vi "Autonomous Independent.vi"   [LabVIEW 2012]
doc: "This VI is called when autonomous begins, and will automatically be terminated when autonomous ends. You can carry out timed or sensor driven robot movement independently without needing to return to the caller."
uses:
  <vilib>/Rock Robotics/WPI/Joystick/WPI_JoystickGetSetRefNum.vi
  Robot Global Data.vi
  <vilib>/Rock Robotics/WPI/RobotDrive/WPI_RobotDriveMecanumDrive_Cartesian.vi
  <vilib>/Rock Robotics/WPI/Solenoid/WPI_SolenoidValue.ctl
  <vilib>/Rock Robotics/WPI/Solenoid/WPI_SolenoidSetEnum.vi
  SubVI/Global 1 (shooter controls).vi
panel:
  # "Be sure to right-click and choose Data Operations>>Make Current Value default if you want to save the array values with the VI"
types:
  T1 = typedef "WPI_SolenoidValue.ctl" = enum16{"Off", "On", "Forward", "Reverse"}
  T2 = enum16{"fire only", "comlex fire 5", "slide left fire", "slide right fire"}
  T3 = typedef "WPI_SolenoidDevRef.ctl" = cluster{"DevStatus":errorcluster, "Solenoid Module":T4, "Forward Solenoid Channel":T5, "Reverse Solenoid Channel":T5}
  T4 = typedef "FPGA_TypedefSolenoidModule.ctl" = enum16{"Solenoid Module 1", "Solenoid Module 2"}
  T5 = typedef "WPI_SolenoidChannel.ctl" = enum8{"Solenoid 1", "Solenoid 2", "Solenoid 3", "Solenoid 4", "Solenoid 5", "Solenoid 6", "Solenoid 7", "Solenoid 8", "Invalid"}
  T6 = typedef "WPI_RobotDriveDevRef.ctl" = cluster{"DevStatus":errorcluster, "Motors[]":T7[], "Square Inputs":bool, "Max Output":dbl, "Isochronous":bool}
  T7 = typedef "WPI_MotorControlDeviceRef.ctl" = cluster{"DeviceStatus":errorcluster, "Type":enum16{"PWM", "CAN"}, "PWM":cluster{"Digital Module":T8, "PWM Channel":T9, "DeadBand":T10}, "CAN":cluster{"Device Number":u8, "Control Mode":T11, "Semaphore":T12, "Max Vout":dbl}, "Invert":bool, "TransformRef":T13, "InvTransformRef":T13}
  T8 = typedef "FPGA_TypedefDigitalModule.ctl" = enum16{"Digital Module 1", "Digital Module 2"}
  T9 = typedef "FPGA_DIOPWMChannel.ctl" = enum8{"PWM 1", "PWM 2", "PWM 3", "PWM 4", "PWM 5", "PWM 6", "PWM 7", "PWM 8", "PWM 9", "PWM 10", "Invalid"}
  T10 = typedef "WPI_PWMDeadband.ctl" = cluster{"Name":string, "maxPositivePwm":i32, "minPositivePwm":i32, "centerPwm":i32, "maxNegativePwm":i32, "minNegativePwm":i32, "angularRange":u16}
  T11 = typedef "WPI_CANJaguar_ControlMode.ctl" = enum8{"Percent VBus", "Current", "Speed", "Position", "Voltage"}
  T12 = typedef "Semaphore RefNum" = refnum<k1>
  T13 = typedef "WPI_PWMTransform_ConPane.ctl" = refnum<vi>
  T14 = typedef "WPI_EncoderDevRef.ctl" = cluster{"DevStatus":errorcluster, "EncoderIndex":T15, "CounterIndex":T16, "DistancePerCount":dbl, "Decoding Type":T17}
  T15 = typedef "FPGA_EncoderIdx.ctl" = enum8{"Enc 0", "Enc 1", "Enc 2", "Enc 3", "Invalid"}
  T16 = typedef "FPGA_CounterCtrSystemIndex.ctl" = enum8{"Ctr 0", "Ctr 1", "Ctr 2", "Ctr 3", "Ctr 4", "Ctr 5", "Ctr 6", "Ctr 7", "Invalid"}
  T17 = typedef "WPI_EncoderType.ctl" = enum16{"1x", "2x", "4x"}
  T18 = typedef "WPI_JoystickDevRef.ctl" = cluster{"Device":T19}
  T19 = typedef "WPI_JoystickDeviceEnum.ctl" = enum16{"USB 1", "USB 2", "USB 3", "USB 4", "Kinect 1", "Kinect 2"}
  T20 = cluster{"axis 1 (x)":dbl, "axis 2 (y)":dbl, "axis 3 (throttle)":dbl, "axis 4":dbl, "axis 5":dbl, "axis 6":dbl}
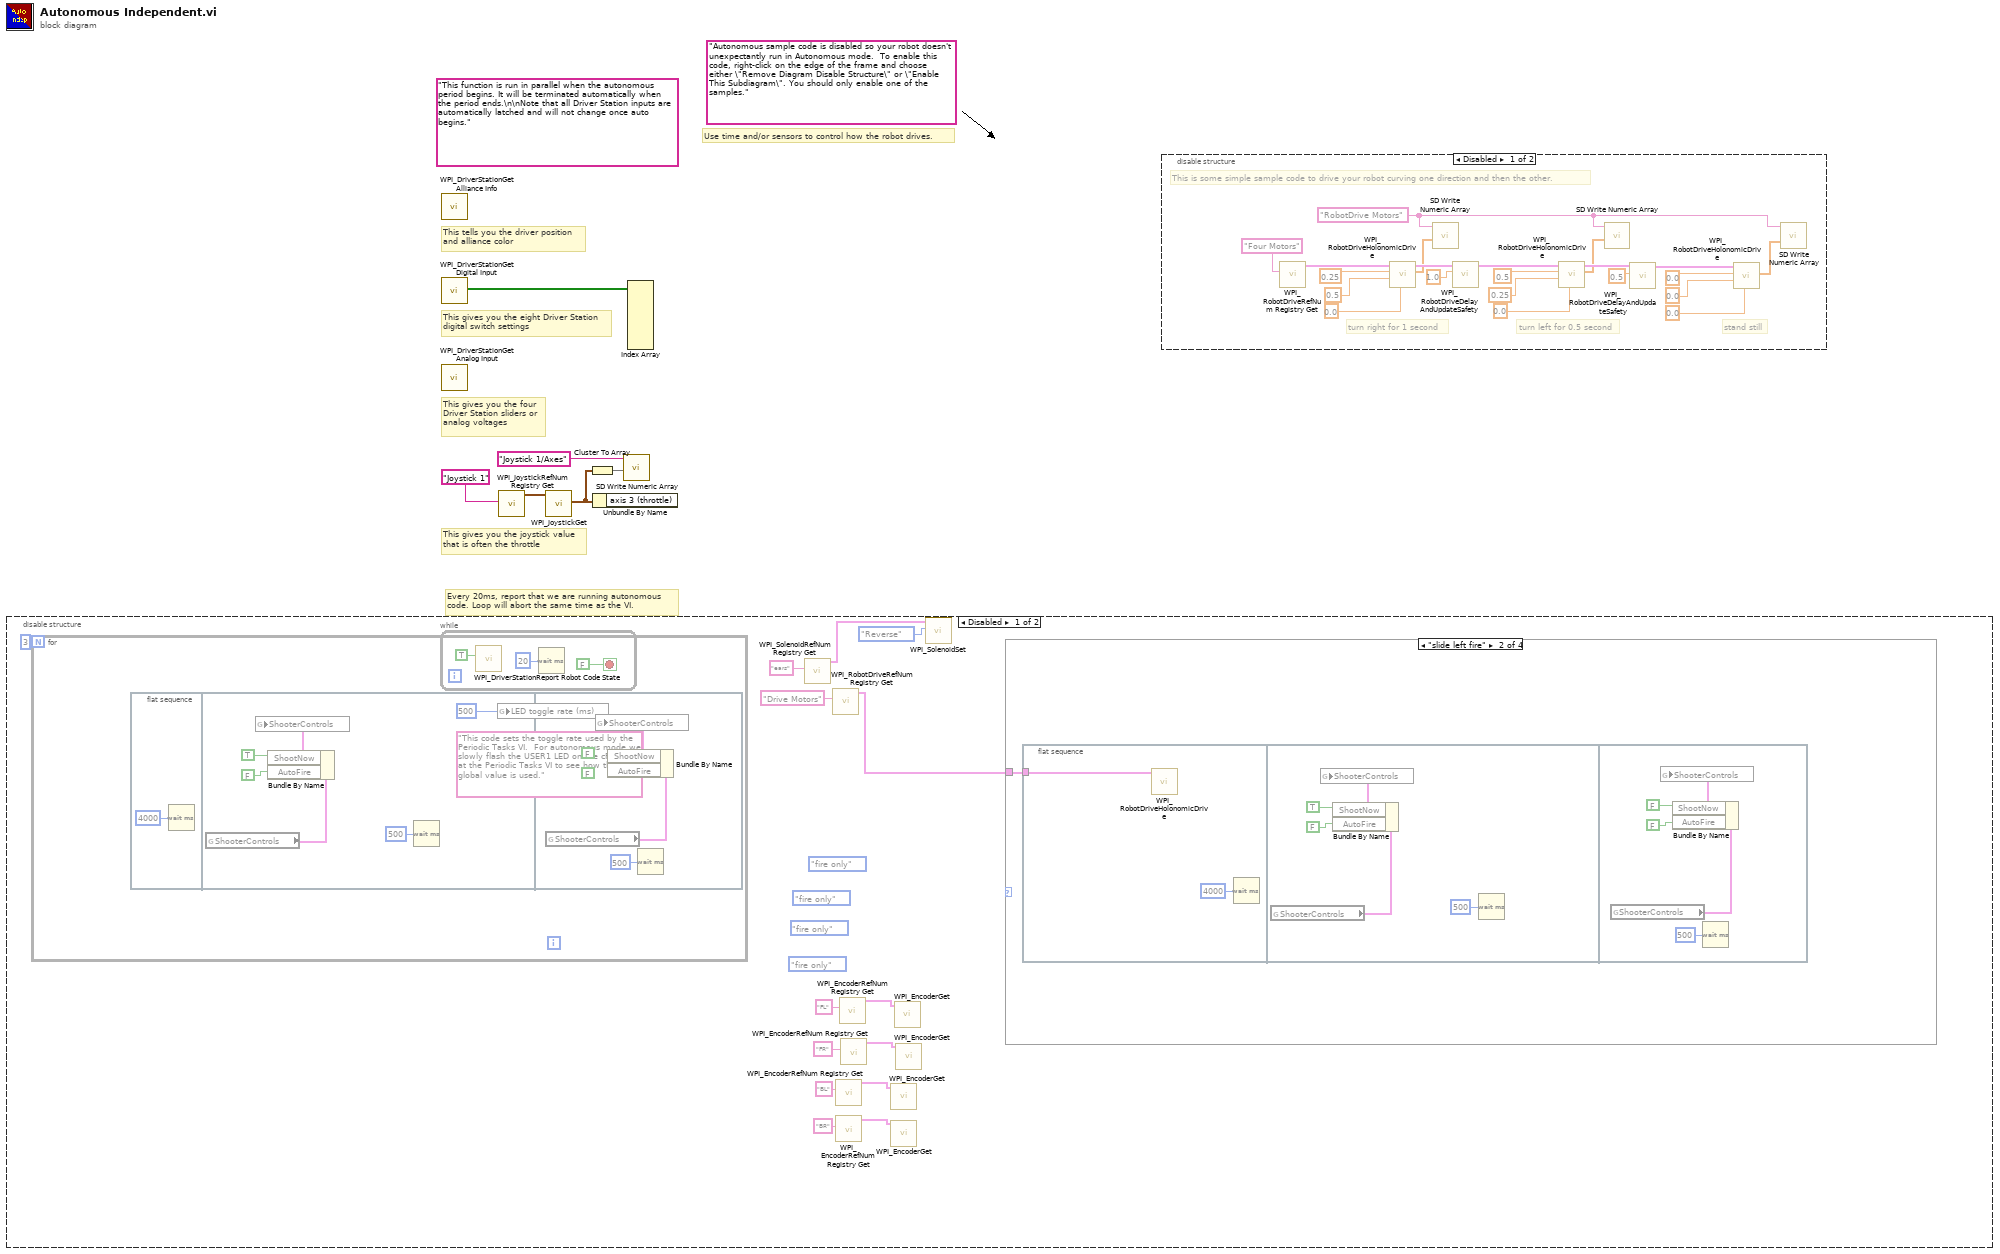
[diagram p0: block diagram]
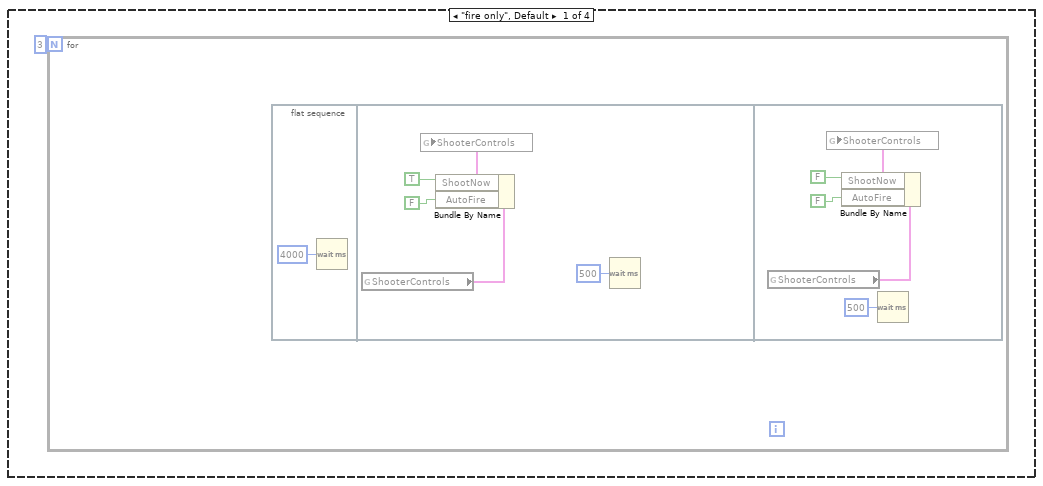
[diagram p2: hidden frame]
diagram:
  (unwired) "Autonomous sample code is disabled so your robot doesn't unexpectantly run in Autonomous mode.  To enable this code, right-click on the edge of the frame and choose either \"Remove Diagram Disable Structure\" or \"Enable This Subdiagram\". You should only enable one of the samples."
  (unwired) "This function is run in parallel when the autonomous period begins. It will be terminated automatically when the period ends.\n\nNote that all Driver Station inputs are automatically latched and will not change once auto begins."
  # "Every 20ms, report that we are running autonomous\ncode. Loop will abort the same time as the VI."
  # "This gives you the joystick value\nthat is often the throttle"
  # "Use time and/or sensors to control how the robot drives."
  # "This tells you the driver position\nand alliance color"
  # "This gives you the eight Driver Station\ndigital switch settings"
  # "This gives you the four\nDriver Station sliders or\nanalog voltages"
  n1 = disable-structure shown="Disabled" {
    frame Disabled {
      (unwired) T2."fire only"
      (unwired) T2."fire only"
      (unwired) T2."fire only"
      (unwired) T2."fire only"
      (unwired) "This code sets the toggle rate used by the Periodic Tasks VI.  For autonomous mode we slowly flash the USER1 LED on the cRIO.  Look at the Periodic Tasks VI to see how this global value is used."
      n2 = for {
        N: 3 -> [_]
        n3 = flat-sequence {
          frame #0 {
            n4 = Wait (ms)(milliseconds to wait=u32 4000) -> ()  [unwired: 1 out]
          }
          frame #1 {
            n5 = global read "Global 1 (shooter controls).vi" "ShooterControls"() -> (w27:cluster{"ShootNow":bool, "AutoFire":bool})
            n6 = Bundle By Name(cluster=w27, "ShootNow"=TRUE, "AutoFire"=FALSE) -> (w26:cluster{"ShootNow":bool, "AutoFire":bool})
            n7 = global write "Global 1 (shooter controls).vi" "ShooterControls"(w26) -> ()
            n8 = Wait (ms)(milliseconds to wait=u32 500) -> ()  [unwired: 1 out]
          }
          frame #2 {
            n9 = global read "Global 1 (shooter controls).vi" "ShooterControls"() -> (w29:cluster{"ShootNow":bool, "AutoFire":bool})
            n10 = Bundle By Name(cluster=w29, "ShootNow"=FALSE, "AutoFire"=FALSE) -> (w30:cluster{"ShootNow":bool, "AutoFire":bool})
            n11 = global write "Global 1 (shooter controls).vi" "ShooterControls"(w30) -> ()
            n12 = Wait (ms)(milliseconds to wait=u32 500) -> ()  [unwired: 1 out]
          }
        }
      }
      n13 = while {
        stop <- FALSE stop-if-true
        n14 = call <vilib>:"WPI_DriverStationReport Robot Code State.vi"("Autonomous"=TRUE) -> ()  [unwired: 10 in, 1 out]
        n15 = Wait (ms)(milliseconds to wait=u32 20) -> ()  [unwired: 1 out]
      }
      n16 = global write "Robot Global Data.vi" "LED toggle rate (ms)"(u32 500 ("LED ms toggle rate")) -> ()
      n17 = call <vilib>:"WPI_SolenoidRefNum Registry Get.vi"("refnum name"="ears") -> ("SolenoidDevRef"=w7:T3)  [unwired: 9 in, 1 out]
      n18 = call <vilib>:"WPI_RobotDriveRefNum Registry Get.vi"("refnum name"="Drive Motors") -> ("RobotDriveDevRef"=w17:T6)  [unwired: 9 in, 1 out]
      n19 = call <vilib>:"WPI_EncoderRefNum Registry Get.vi"("refnum name"="BL") -> ("EncoderDevRef"=w14:T14)  [unwired: 9 in, 1 out]
      n20 = call <vilib>:"WPI_EncoderRefNum Registry Get.vi"("refnum name"="BR") -> ("EncoderDevRef"=w13:T14)  [unwired: 9 in, 1 out]
      n21 = call <vilib>:"WPI_EncoderRefNum Registry Get.vi"("refnum name"="FL") -> ("EncoderDevRef"=w16:T14)  [unwired: 9 in, 1 out]
      n22 = call <vilib>:"WPI_EncoderRefNum Registry Get.vi"("refnum name"="FR") -> ("EncoderDevRef"=w15:T14)  [unwired: 9 in, 1 out]
      n23 = call <vilib>:"WPI_EncoderGet.vi"("EncoderDevRef"=w14) -> ()  [unwired: 5 in, 6 out]
      n24 = call <vilib>:"WPI_EncoderGet.vi"("EncoderDevRef"=w13) -> ()  [unwired: 5 in, 6 out]
      n25 = call <vilib>:"WPI_EncoderGet.vi"("EncoderDevRef"=w16) -> ()  [unwired: 5 in, 6 out]
      n26 = call <vilib>:"WPI_EncoderGet.vi"("EncoderDevRef"=w15) -> ()  [unwired: 5 in, 6 out]
      n27 = call-poly <vilib>:"WPI_SolenoidSet.vi"("Value"=WPI_SolenoidValue."Reverse", "SolenoidDevRef"=w7) -> ()  [unwired: 8 in, 2 out]
      n28 = case shown="\"slide left fire\"" {
        selector: _ -> [_ _ _ _]
        tunnel: w17 -> [_ w45 _ _]
        frame "fire only", Default {
          n29 = for {
            N: 3 -> [_]
            n30 = flat-sequence {
              frame #0 {
                n31 = Wait (ms)(milliseconds to wait=u32 4000) -> ()  [unwired: 1 out]
              }
              frame #1 {
                n32 = global read "Global 1 (shooter controls).vi" "ShooterControls"() -> (w39:cluster{"ShootNow":bool, "AutoFire":bool})
                n33 = Bundle By Name(cluster=w39, "ShootNow"=TRUE, "AutoFire"=FALSE) -> (w38:cluster{"ShootNow":bool, "AutoFire":bool})
                n34 = global write "Global 1 (shooter controls).vi" "ShooterControls"(w38) -> ()
                n35 = Wait (ms)(milliseconds to wait=u32 500) -> ()  [unwired: 1 out]
              }
              frame #2 {
                n36 = global read "Global 1 (shooter controls).vi" "ShooterControls"() -> (w41:cluster{"ShootNow":bool, "AutoFire":bool})
                n37 = Bundle By Name(cluster=w41, "ShootNow"=FALSE, "AutoFire"=FALSE) -> (w42:cluster{"ShootNow":bool, "AutoFire":bool})
                n38 = global write "Global 1 (shooter controls).vi" "ShooterControls"(w42) -> ()
                n39 = Wait (ms)(milliseconds to wait=u32 500) -> ()  [unwired: 1 out]
              }
            }
          }
        }
        frame "slide left fire" {
          n40 = flat-sequence {
            tunnel: w45 -> [w46]
            frame #0 {
              n41 = call-poly <vilib>:"WPI_RobotDriveHolonomicDrive.vi"("RobotDriveDevRef"=w46) -> ()  [unwired: 8 in, 3 out]
              n42 = Wait (ms)(milliseconds to wait=u32 4000) -> ()  [unwired: 1 out]
            }
            frame #1 {
              n43 = global read "Global 1 (shooter controls).vi" "ShooterControls"() -> (w52:cluster{"ShootNow":bool, "AutoFire":bool})
              n44 = Bundle By Name(cluster=w52, "ShootNow"=TRUE, "AutoFire"=FALSE) -> (w51:cluster{"ShootNow":bool, "AutoFire":bool})
              n45 = global write "Global 1 (shooter controls).vi" "ShooterControls"(w51) -> ()
              n46 = Wait (ms)(milliseconds to wait=u32 500) -> ()  [unwired: 1 out]
            }
            frame #2 {
              n47 = global read "Global 1 (shooter controls).vi" "ShooterControls"() -> (w54:cluster{"ShootNow":bool, "AutoFire":bool})
              n48 = Bundle By Name(cluster=w54, "ShootNow"=FALSE, "AutoFire"=FALSE) -> (w55:cluster{"ShootNow":bool, "AutoFire":bool})
              n49 = global write "Global 1 (shooter controls).vi" "ShooterControls"(w55) -> ()
              n50 = Wait (ms)(milliseconds to wait=u32 500) -> ()  [unwired: 1 out]
            }
          }
        }
        frame "slide right fire" {
        }
        frame "comlex fire 5" {
        }
      }
    }
    frame Enabled {
    }
  }
  n51 = call <vilib>:"WPI_DriverStationGet Alliance Info.vi"() -> ()  [unwired: 12 out]
  n52 = call <vilib>:"WPI_DriverStationGet Digital Input.vi"() -> ("Driver Station Digital Input (1-8)"=w6:bool[])  [unwired: 11 out]
  n53 = call <vilib>:"WPI_DriverStationGet Analog Input.vi"() -> ()  [unwired: 12 out]
  n54 = call <vilib>:"WPI_JoystickRefNum Registry Get.vi"("refnum name"="Joystick 1") -> ("JoystickDevRef"=w4:T18)  [unwired: 1 in, 9 out]
  n55 = call <vilib>:"WPI_JoystickGet.vi"("JoystickDevRef"=w4) -> ("Axes"=w2:T20)  [unwired: 1 in, 5 out]
  n56 = Cluster To Array(cluster=w2) -> (array=w3:dbl[])
  n57 = Unbundle By Name(w2) -> ()  [unwired: 1 out]
  n58 = call <vilib>:"SD Write Numeric Array.vi"("Numeric Array"=w3, "Name"="Joystick 1/Axes") -> ()  [unwired: 8 in, 2 out]
  n59 = Index Array(array=w6) -> ()  [unwired: 8 in, 8 out]
  n60 = disable-structure shown="Disabled" {
    frame Disabled {
      w64 = "RobotDrive Motors" ("Name")
      # "This is some simple sample code to drive your robot curving one direction and then the other."
      # "stand still"
      # "turn left for 0.5 second"
      # "turn right for 1 second"
      n61 = call <vilib>:"WPI_RobotDriveRefNum Registry Get.vi"("refnum name"="Four Motors") -> ("RobotDriveDevRef"=w68:T6)  [unwired: 1 in, 9 out]
      n62 = call-poly <vilib>:"WPI_RobotDriveHolonomicDrive.vi"("Rotation"=0.0, "Y"=0.5 ("X axis value"), "X"=0.25 ("X axis value"), "RobotDriveDevRef"=w68) -> ("Motor Values"=w67:dbl[], "RobotDriveDevRef"=w75:T6)  [unwired: 5 in, 1 out]
      n63 = call <vilib>:"SD Write Numeric Array.vi"("Numeric Array"=w67, "Name"=w64) -> ()  [unwired: 8 in, 2 out]
      n64 = call <vilib>:"WPI_RobotDriveDelayAndUpdateSafety.vi"("Delay (s)"=1.0, "RobotDriveDevRef"=w75) -> ("RobotDriveDevRef 2"=w74:T6)  [unwired: 8 in, 1 out]
      n65 = call-poly <vilib>:"WPI_RobotDriveHolonomicDrive.vi"("Rotation"=0.0, "Y"=0.25 ("X axis value"), "X"=0.5 ("X axis value"), "RobotDriveDevRef"=w74) -> ("Motor Values"=w66:dbl[], "RobotDriveDevRef"=w73:T6)  [unwired: 5 in, 1 out]
      n66 = call <vilib>:"SD Write Numeric Array.vi"("Numeric Array"=w66, "Name"=w64) -> ()  [unwired: 8 in, 2 out]
      n67 = call <vilib>:"WPI_RobotDriveDelayAndUpdateSafety.vi"("Delay (s)"=0.5, "RobotDriveDevRef"=w73) -> ("RobotDriveDevRef 2"=w72:T6)  [unwired: 8 in, 1 out]
      n68 = call-poly <vilib>:"WPI_RobotDriveHolonomicDrive.vi"("Rotation"=0.0 ("X axis value"), "Y"=0.0 ("X axis value"), "X"=0.0 ("X axis value"), "RobotDriveDevRef"=w72) -> ("Motor Values"=w65:dbl[])  [unwired: 5 in, 2 out]
      n69 = call <vilib>:"SD Write Numeric Array.vi"("Numeric Array"=w65, "Name"=w64) -> ()  [unwired: 8 in, 2 out]
    }
    frame Enabled {
    }
  }
